vi "Planet_UserInterface.vi"(8 "error in":errorcluster, 9 "Number of it":i32, 11 "Conf":T1) -> (0 "error out":errorcluster, 3 "Exit?":bool)   [LabVIEW 2021]
uses:
  Typedefs/Axis.ctl
  Typedefs/ConfCluster.ctl
  Typedefs/All_Queues.ctl
  Typedefs/DataToUserInterface.ctl
  Typedefs/PropertyUserChange.ctl
  Typedefs/PropertiesRead_TDM.ctl
  Typedefs/Start_End.ctl
  Typedefs/OrderAnalysis.ctl
  Typedefs/MeassurementMode.ctl
  Typedefs/PropertiesOrderAnalysis.ctl
  Typedefs/AllDataToAnal.ctl
  Typedefs/PlanetInfo.ctl
  Typedefs/Detected peaks.ctl
  Typedefs/Referencias.ctl
  Typedefs/OpenClose.ctl
  Typedefs/DataToUI.ctl
  Typedefs/Results.ctl
panel:
  in  "Btn_Alarm":bool
  in  "Lock":bool
  in  "Stop":bool
  in  "Exit":bool
  in  "Btn_Mesh":bool
  in  "Btn_Order":bool
  in  "Btn_Spec":bool
  in  "Btn_Main":bool
  in  "Start":bool
  in  "Results":T6(tab)
  out "Vibration signals":waveform(dbl)[](graph)
  out "Speed profile":cluster{"time [s]":dbl[], "speed [RPM]":dbl[]}(graph)
  out "Input - Power Spectrum":cluster{"f0":dbl, "df":dbl, "magnitude":dbl[]}[](graph)
  out "Output - Power Spectrum":cluster{"f0":dbl, "df":dbl, "magnitude":dbl[]}[](graph)
  out "Input - Order power spectrum":T7(graph)
  out "Input - Actual max order":dbl
  out "Output - Order power spectrum":T7(graph)
  out "Output - Actual max order":dbl
  out "Input - fz":dbl[](graph) caption="Output - fz"
  out "Output_mean":dbl format="%0.2f"
  out "Output_std":dbl format="%0.2f"
  out "Input_mean":dbl format="%0.2f"
  out "WejścieInput":dbl format="%0.2f"
  out "Output - fz":dbl[](graph) caption="Input - fz"
  in  "Axis":T8 items=["X", "Y", "Z"]
  in  "Exceedances":i32(listbox)
  in  "MainSettings":enum32{"Page 1"}(tab)
  in  "averaging mode":u16(ring) items=["No averaging", "Vector averaging", "RMS averaging", "Peak hold"]
  in  "order resolution":dbl=0.1 min=0.0 format="%.3f"
  in  "window type":T9(ring)=enum."Hanning"
  in  "dB on":bool=TRUE
  in  "max order to analyze":dbl=32.0
  in  "Sample rate":i64=51200
  in  "File path":path
  in  "Channels":tag
  in  "Sample mode":i32(ring)=10123 items=["Finite Samples"=10178, "Continuous Samples"=10123, "Hardware Timed Single Point"=12522]
  in  "Terminal conf":i32(ring)=12529 items=["Default"=-1, "RSE"=10083, "NRSE"=10078, "Differential"=10106, "Pseudodifferential"=12529]
  in  "Multiple of Frequency":i32=3
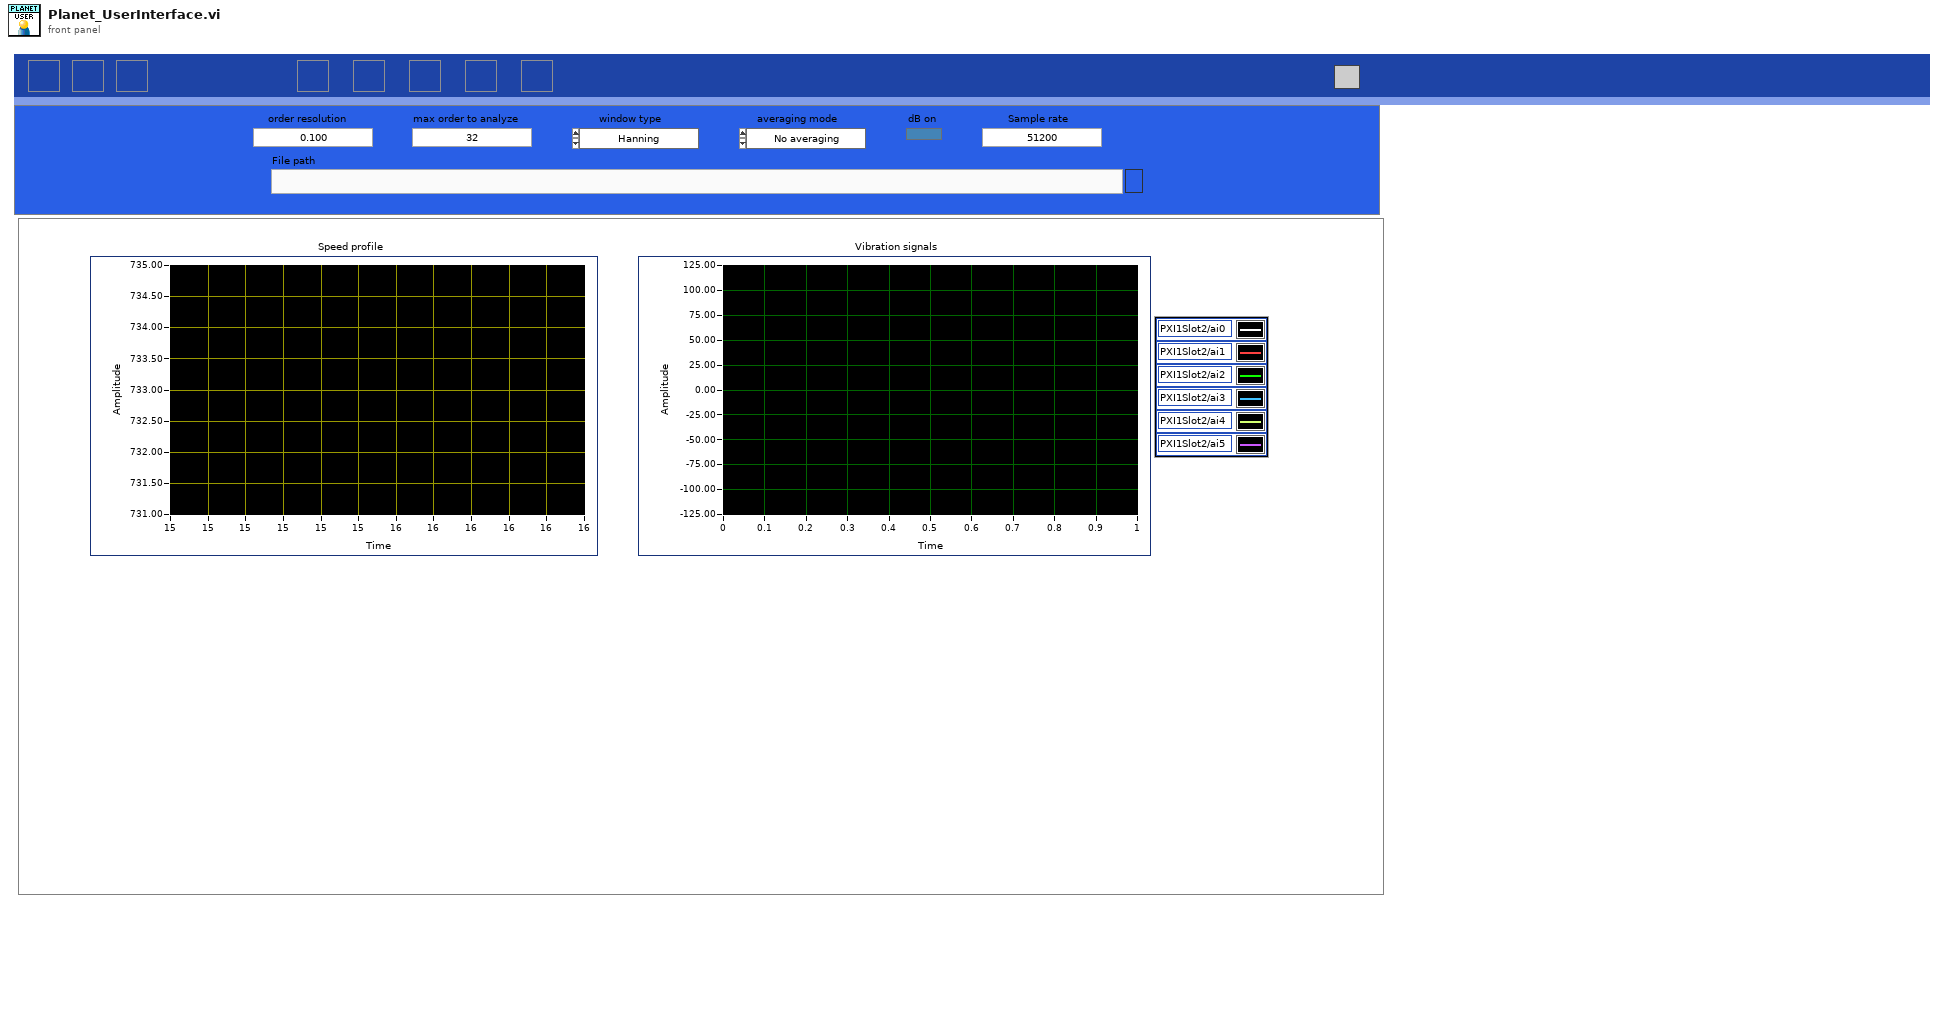
[diagram p1: front panel]
types:
  T1 = typedef "ConfCluster.ctl" = cluster{"Plik?":bool, "Queues":T2, "NewFile":path, "AllDataToAnal":T3}
  T2 = typedef "All_Queues.ctl" = cluster{"User Event":refnum<user-event>, "ToAcq":refnum<queue>, "ToOA":refnum<queue>}
  T3 = typedef "AllDataToAnal.ctl" = cluster{"PlanetInfo":T4, "Referencia":T5[][], "Ref?":bool}
  T4 = typedef "PlanetInfo.ctl" = cluster{"Ms":dbl, "Np":dbl, "Ns":dbl, "Nr":dbl}
  T5 = typedef "Detected peaks.ctl" = cluster{"detected frequency":dbl, "detected amplitude":dbl}
  T6 = enum32{"Main", "PowerSpectrum", "Order analysis", "Mesh Frequency", "Alarms"}
  T7 = cluster{"order 0":dbl, "delta order":dbl, "magnitude":dbl[]}[]
  T8 = typedef "Axis.ctl" = u16
  T9 = enum16{"None", "Hanning", "Hamming", "Blackman-Harris", "Exact Blackman", "Blackman", "Flat Top", "4 Term B-Harris", "7 Term B-Harris", "Low Sidelobe", "Gaussian"}
  T10 = typedef "Referencias.ctl" = cluster{"MainSettings":refnum<vi>, "Results":refnum<vi>, "FirstLineSettings":refnum<vi>[], "FromFile":refnum<vi>, "Meassurement":refnum<vi>[], "MainGraphs":refnum<vi>[], "OAGraphs":refnum<vi>[], "OA_MaxOrder":refnum<vi>[], "PSGraphs":refnum<vi>[], "Fz":refnum<vi>[], "mean_std":refnum<vi>[], "Btn":refnum<vi>[], "This VI":refnum<vi>, "Przekroczenia":refnum<vi>, "Axis":refnum<vi>, "Main_Btn":refnum<vi>[]}
  T11 = typedef "OpenClose.ctl" = enum16{"Close", "Open"}
  T12 = typedef "PropertiesRead_TDM.ctl" = cluster{"Start/End":T13, "stop":bool, "file path":path, "OrderAnalysis":T14, "Meassurement Mode":T15}
  T13 = typedef "Start_End.ctl" = enum16{"Start", "End"}
  T14 = typedef "OrderAnalysis.ctl" = cluster{"dB on":bool, "window type":u32, "max order to analyze":dbl, "order resolution":dbl, "Axis":T8, "Sample rate":i64, "Save?":bool, "Multiple_Frequency":i32, "averaging mode":enum16{"No averaging", "Vector averaging", "RMS averaging", "Peak hold"}}
  T15 = typedef "MeassurementMode.ctl" = cluster{"Sample mode":i32, "Terminal conf":i32, "Channels":tag}
  T16 = typedef "DataToUI.ctl" = cluster{"Speed profile":cluster{"time [s]":dbl[], "speed [RPM]":dbl[]}, "Results":T17[], "Vibration signals":waveform(dbl)[]}
  T17 = typedef "Results.ctl" = cluster{"Power Spectrum / PSD":cluster{"f0":dbl, "df":dbl, "magnitude":dbl[]}[], "Order power spectra":cluster{"order 0":dbl, "delta order":dbl, "magnitude":dbl[]}[], "Actual max order":dbl, "Mesh_Freq":dbl[], "Detected peaks":T5[][], "Alarm?":bool[], "Exceed":string[][], "Mesh_mean":dbl, "Mesh_std":dbl}
  T18 = typedef "PropertyUserChange.ctl" = enum16{"Default", "Results", "Start", "Save", "CanalNames"}
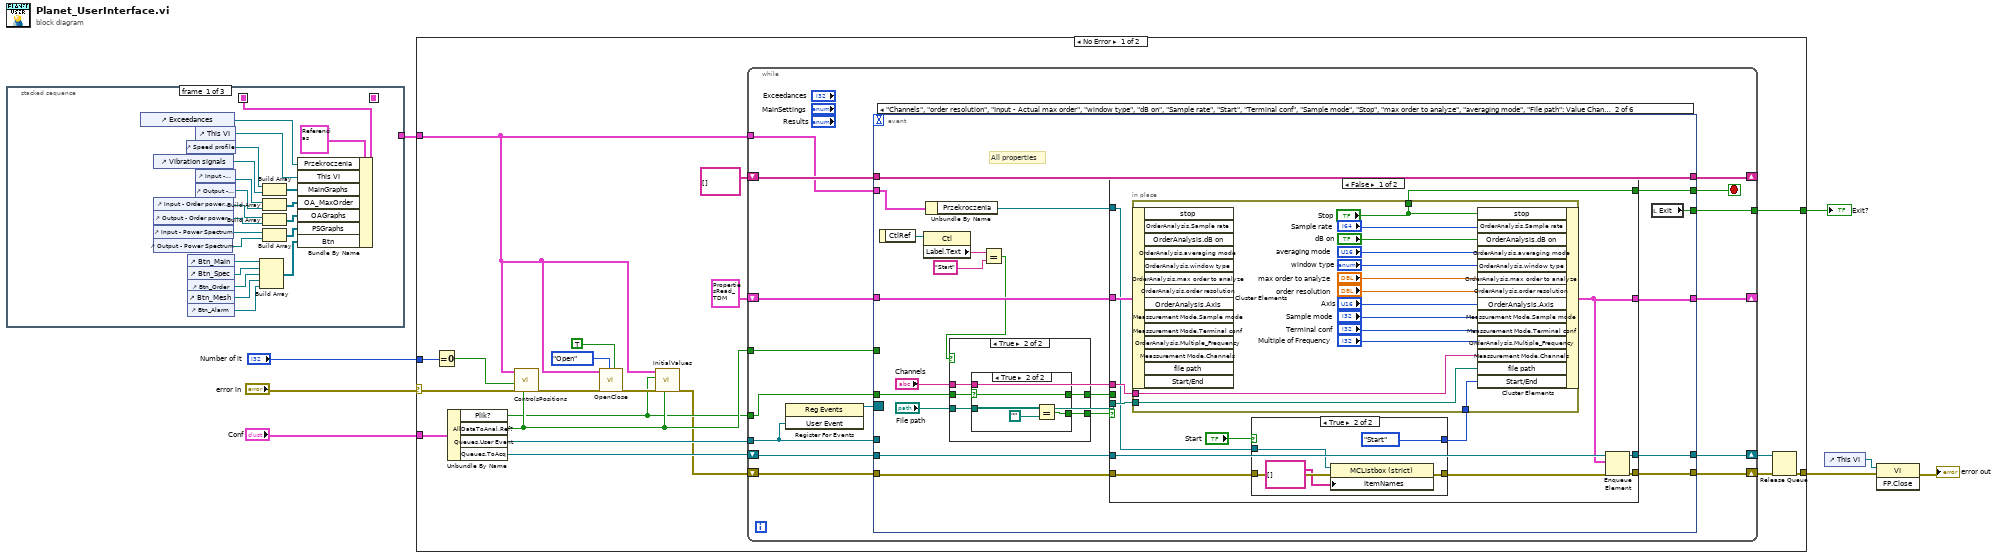
[diagram p0: block diagram]
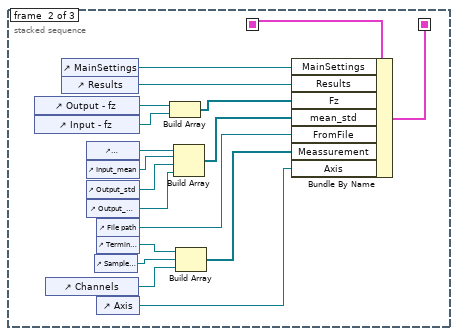
[diagram p2: hidden frame]
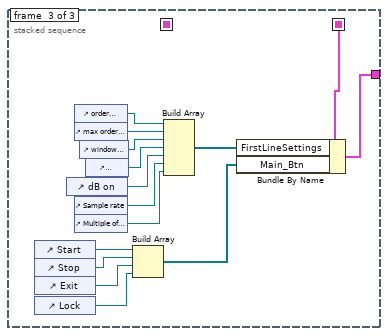
[diagram p3: hidden frame]
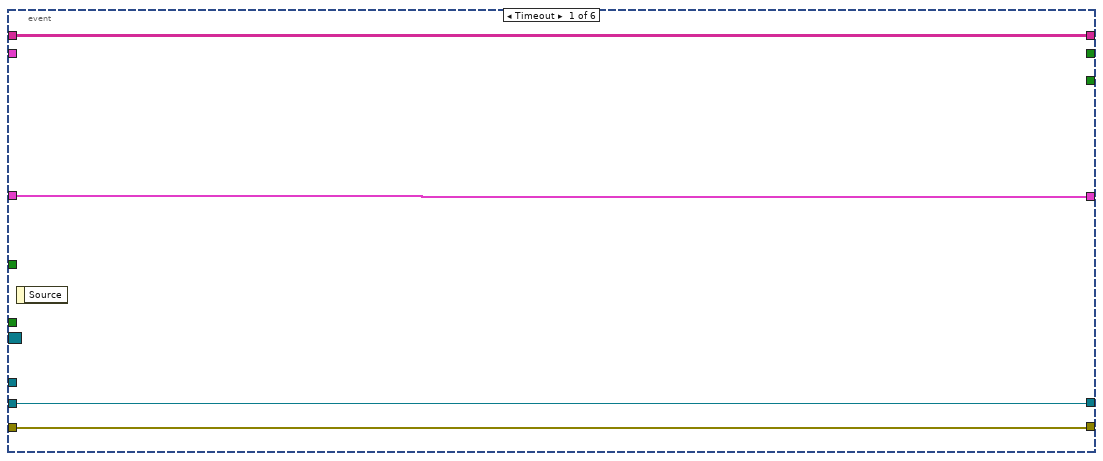
[diagram p4: hidden frame]
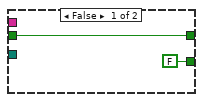
[diagram p5: hidden frame]
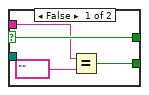
[diagram p6: hidden frame]
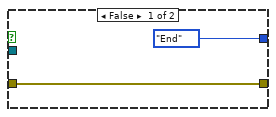
[diagram p7: hidden frame]
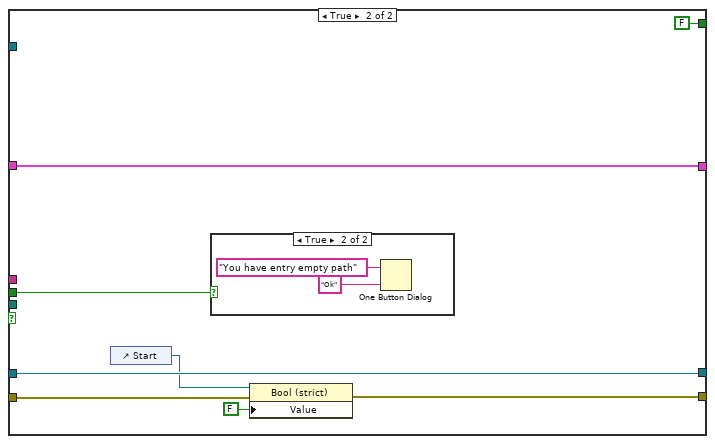
[diagram p8: hidden frame]
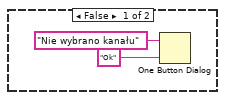
[diagram p9: hidden frame]
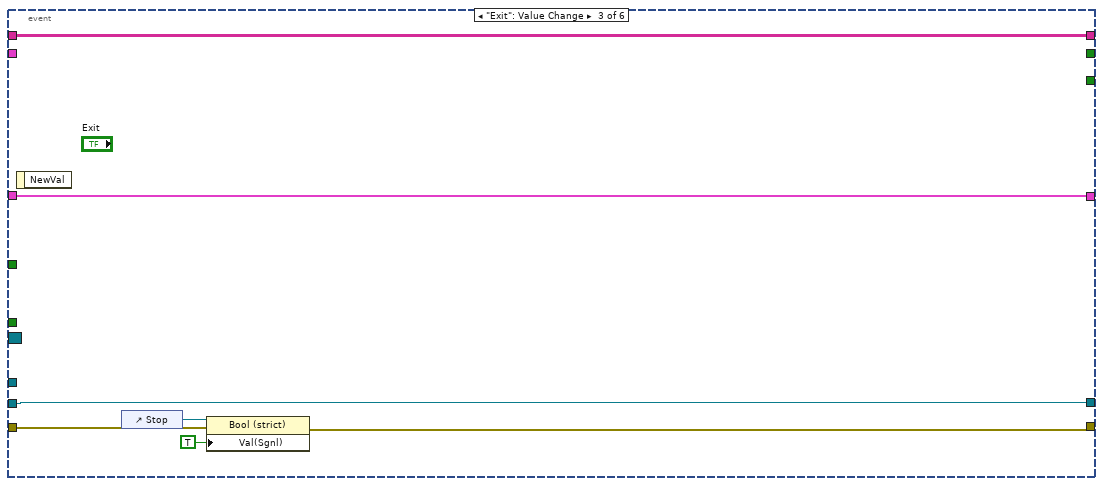
[diagram p10: hidden frame]
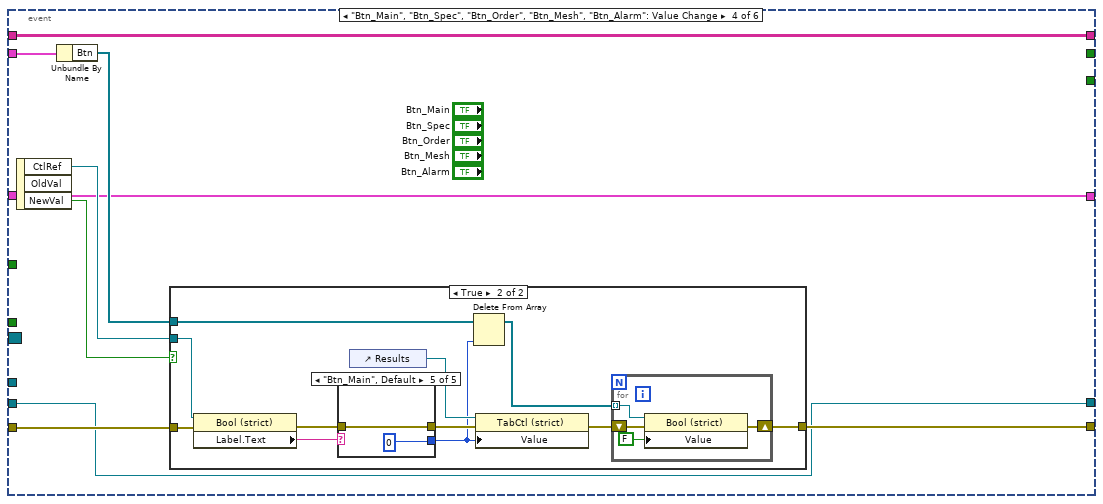
[diagram p11: hidden frame]
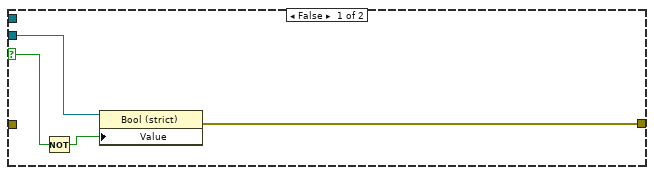
[diagram p12: hidden frame]
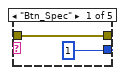
[diagram p13: hidden frame]
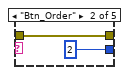
[diagram p14: hidden frame]
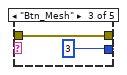
[diagram p15: hidden frame]
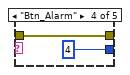
[diagram p16: hidden frame]
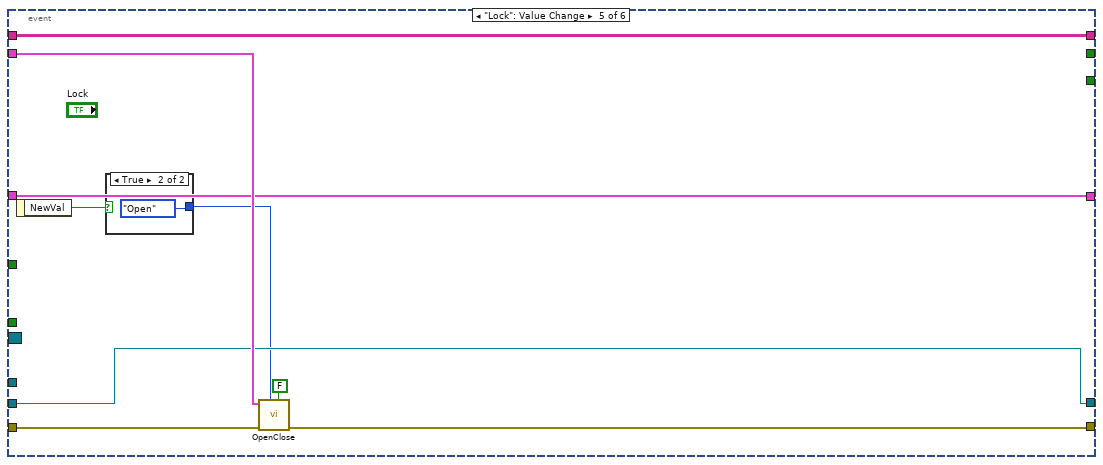
[diagram p17: hidden frame]
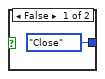
[diagram p18: hidden frame]
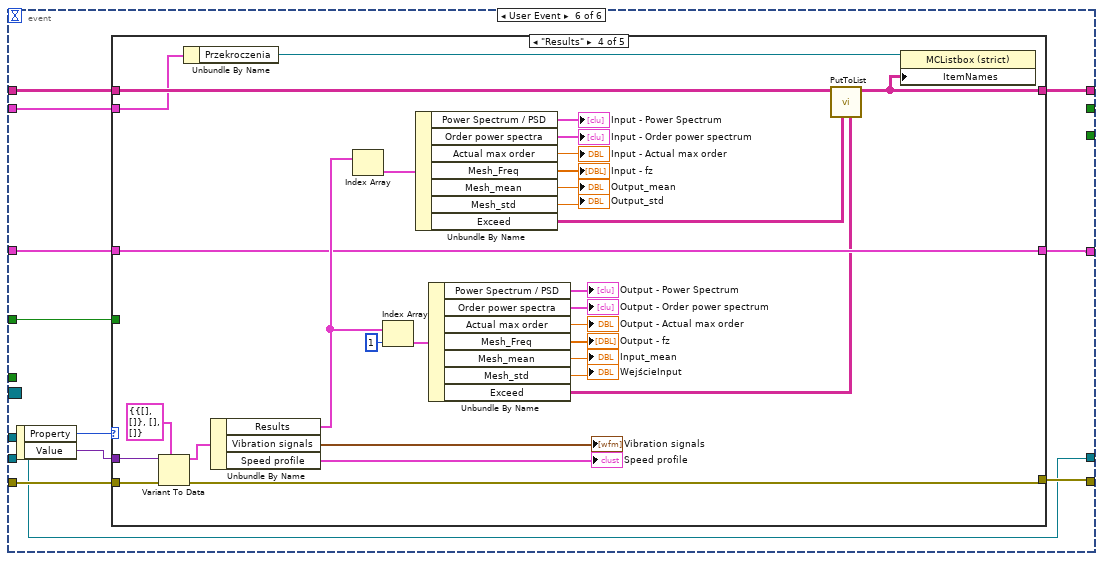
[diagram p19: hidden frame]
diagram:
  n1 = stacked-sequence {
    seq-local: [w15 _ _] -> [_ w33 _]
    seq-local: [_ w31 _] -> [_ _ w51]
    tunnel: [_ _ w50] -> w1
    frame #0 {
      n2 = control-ref of="Exceedances"() -> (w21:refnum<vi>)
      n3 = control-ref of="Output - Power Spectrum"() -> (w30:refnum<vi>)
      n4 = control-ref of="Vibration signals"() -> (w24:refnum<vi>)
      n5 = control-ref of="Input - Order power spectrum"() -> (w27:refnum<vi>)
      n6 = control-ref of="Output - Order power spectrum"() -> (w28:refnum<vi>)
      n7 = control-ref of="Input - Power Spectrum"() -> (w29:refnum<vi>)
      n8 = control-ref of="Speed profile"() -> (w23:refnum<vi>)
      n9 = control-ref of="Btn_Main"() -> (w10:refnum<vi>)
      n10 = control-ref of="Btn_Spec"() -> (w11:refnum<vi>)
      n11 = control-ref of="Btn_Order"() -> (w12:refnum<vi>)
      n12 = control-ref of="Btn_Mesh"() -> (w13:refnum<vi>)
      n13 = control-ref of="Btn_Alarm"() -> (w14:refnum<vi>)
      n14 = control-ref of="This VI"() -> (w20:refnum<vi>)
      n15 = control-ref of="Input - Actual max order"() -> (w25:refnum<vi>)
      n16 = control-ref of="Output - Actual max order"() -> (w26:refnum<vi>)
      n17 = Build Array(w10, w11, w12, w13, w14) -> (w9:refnum<vi>[])
      n18 = Build Array(w23, w24) -> (w19:refnum<vi>[])
      n19 = Build Array(w25, w26) -> (w18:refnum<vi>[])
      n20 = Build Array(w27, w28) -> (w17:refnum<vi>[])
      n21 = Build Array(w29, w30) -> (w16:refnum<vi>[])
      n22 = Bundle By Name(cluster=T10 {"MainSettings"=refnum, "Results"=refnum, "FirstLineSettings"=[], "FromFile"=refnum, "Meassurement"=[], "MainGraphs"=[], "OAGraphs"=[], "OA_MaxOrder"=[], "PSGraphs"=[], "Fz"=[], "mean_std"=[], "Btn"=[], "This VI"=refnum, "Przekroczenia"=refnum, "Axis"=refnum, "Main_Btn"=[]} ("References"), "Przekroczenia"=w21, "This VI"=w20, "MainGraphs"=w19, "OA_MaxOrder"=w18, "OAGraphs"=w17, "PSGraphs"=w16, "Btn"=w9) -> (w15:T10)
    }
    frame #1 {
      n23 = control-ref of="Output - fz"() -> (w48:refnum<vi>)
      n24 = control-ref of="Input - fz"() -> (w43:refnum<vi>)
      n25 = control-ref of="Channels"() -> (w40:refnum<vi>)
      n26 = control-ref of="MainSettings"() -> (w39:refnum<vi>)
      n27 = control-ref of="Results"() -> (w38:refnum<vi>)
      n28 = control-ref of="WejścieInput"() -> (w44:refnum<vi>)
      n29 = control-ref of="Input_mean"() -> (w45:refnum<vi>)
      n30 = control-ref of="Output_std"() -> (w46:refnum<vi>)
      n31 = control-ref of="Output_mean"() -> (w47:refnum<vi>)
      n32 = control-ref of="Sample mode"() -> (w42:refnum<vi>)
      n33 = control-ref of="File path"() -> (w35:refnum<vi>)
      n34 = control-ref of="Terminal conf"() -> (w41:refnum<vi>)
      n35 = control-ref of="Axis"() -> (w32:refnum<vi>)
      n36 = Build Array(w48, w43) -> (w37:refnum<vi>[])
      n37 = Build Array(w44, w45, w46, w47) -> (w36:refnum<vi>[])
      n38 = Build Array(w41, w42, w40) -> (w34:refnum<vi>[])
      n39 = Bundle By Name(cluster=w33, "MainSettings"=w39, "Results"=w38, "Fz"=w37, "mean_std"=w36, "FromFile"=w35, "Meassurement"=w34, "Axis"=w32) -> (w31:T10)
    }
    frame #2 {
      n40 = control-ref of="Start"() -> (w60:refnum<vi>)
      n41 = control-ref of="Stop"() -> (w61:refnum<vi>)
      n42 = control-ref of="Exit"() -> (w49:refnum<vi>)
      n43 = control-ref of="Lock"() -> (w62:refnum<vi>)
      n44 = control-ref of="dB on"() -> (w58:refnum<vi>)
      n45 = control-ref of="order resolution"() -> (w54:refnum<vi>)
      n46 = control-ref of="max order to analyze"() -> (w55:refnum<vi>)
      n47 = control-ref of="Sample rate"() -> (w59:refnum<vi>)
      n48 = control-ref of="Multiple of Frequency"() -> (w63:refnum<vi>)
      n49 = control-ref of="window type"() -> (w56:refnum<vi>)
      n50 = control-ref of="averaging mode"() -> (w57:refnum<vi>)
      n51 = Build Array(w60, w61, w49, w62) -> (w52:refnum<vi>[])
      n52 = Build Array(w54, w55, w56, w57, w58, w59, w63) -> (w53:refnum<vi>[])
      n53 = Bundle By Name(cluster=w51, "FirstLineSettings"=w53, "Main_Btn"=w52) -> (w50:T10)
    }
  }
  n54 = case shown="No Error" "error in" {
    selector: "error in" -> [w71 w338]
    tunnel: [w78 _] -> w8
    tunnel: "Conf" -> [w72 _]
    tunnel: [w70 w338] -> w5
    tunnel: "Number of it" -> [w65 _]
    tunnel: w1 -> [w67 _]
    frame No Error {
      n55 = Equal To 0?(x=w65) -> (x = 0?=w64:bool)
      n56 = Unbundle By Name(w72) -> ("Plik?"=w68:bool, "AllDataToAnal.Ref?"=w73:bool, "Queues.User Event"=w80:refnum<user-event>, "Queues.ToAcq"=w81:refnum<queue>)
      n57 = call "ControlsPositions.vi"("Ref?"=w73, "error in (no error)"=w71, "Boolean"=w64, "Referencia"=w67) -> ("error out"=w76:errorcluster)  [unwired: 7 in]
      n58 = call "OpenClose.vi"("FastOpen?"=TRUE, "Open/Close"=OpenClose."Open", "error in"=w76, "References"=w67) -> ("error out"=w75:errorcluster)  [unwired: 7 in]
      n59 = call "InitialValues.vi"("Ref?"=w73, "error in (no error)"=w75, "Plik?"=w68, "References"=w67) -> ("error out"=w66:errorcluster)  [unwired: 7 in]
      n60 = while {
        shift-right: [w94] -> w83
        shift-left: w81 -> [w96]
        shift-right: [w93] -> w82
        shift-left: w66 -> [w95]
        shift-right: [w97] -> _
        shift-left: T12 {"Start/End"=enum."End", "stop"=FALSE, "file path"=path "", "OrderAnalysis"={"dB on"=TRUE, "window type"=1, "max order to analyze"=32.0, "order resolution"=0.1, "Axis"=0, "Sample rate"=5000, "Save?"=FALSE, "Multiple_Frequency"=3, "averaging mode"=enum."No averaging"}, "Meassurement Mode"={"Sample mode"=10123, "Terminal conf"=12529, "Channels"=""}} -> [w98]
        tunnel: w80 -> [w90]
        tunnel: [w89] -> w78
        shift-right: [w87] -> _
        shift-left: string[][] [] ("Next") -> [w88]
        tunnel: w73 -> [w86]
        tunnel: w68 -> [w85]
        tunnel: w67 -> [w84]
        stop <- w92 stop-if-true
        n61 = register-events(w90) -> (reference out=w91:refnum<event-registration>)  [unwired: 2 in, 1 out]
        n62 = event shown="[1] \"Channels\", \"order resolution\", \"Input - Actual max order\", \"window type\", \"dB on\", \"Sample rate\", \"Start\", \"Terminal conf\", \"Sample mode\", \"Stop\", \"max order to analyze\", \"averaging mode\", \"File path\": Value Change" {
          selector: w91 -> [_ _ _ _ _ _]
          dyn-events: _ -> [_ _ _ _ _ _]
          timeout: _ -> [_ _ _ _ _ _]
          tunnel: w98 -> [w102 w122 w189 w193 w232 w245]
          tunnel: [w102 w117 w189 w193 w232 w244] -> w97
          tunnel: w96 -> [w101 w121 w187 w192 w233 w246]
          tunnel: w95 -> [w100 w120 w190 w194 w237 w249]
          tunnel: [w101 w119 w187 w192 w233 w246] -> w94
          tunnel: [w100 w118 w188 w195 w235 w248] -> w93
          tunnel: [_ w115 _ _ _ _] -> w92
          tunnel: w90 -> [_ _ _ _ _ _]
          tunnel: w84 -> [_ w108 _ w197 w236 w240]
          tunnel: [_ w114 _ _ _ _] -> w89
          tunnel: w88 -> [w99 w116 w184 w191 w229 w243]
          tunnel: [w99 w116 w184 w191 w229 w242] -> w87
          tunnel: w86 -> [_ _ _ _ _ w241]
          tunnel: w85 -> [_ w112 _ _ _ _]
          event Timeout {
            n63 = event-data() -> ()  [unwired: 1 in, 1 out]
          }
          event "Channels", "order resolution", "Input - Actual max order", "window type", "dB on", "Sample rate", "Start", "Terminal conf", "Sample mode", "Stop", "max order to analyze", "averaging mode", "File path": Value Change {
            # "All properties"
            n64 = event-data() -> ("CtlRef"=w106:refnum<vi>)  [unwired: 1 in]
            n65 = property class="Ctl"(reference=w106) -> ("Label.Text"=w105:string)  [unwired: 1 in, 2 out]
            n66 = Unbundle By Name(w108) -> ("Przekroczenia"=w107:refnum<vi>)
            n67 = Equal?(x=w105, y="Start") -> (x = y?=w103:bool)
            n68 = case shown="True" w103 {
              tunnel: [FALSE w129] -> w113
              tunnel: w112 -> [w124 w128]
              tunnel: "Channels" -> [_ w127]
              tunnel: "File path" -> [_ w126]
              tunnel: [w124 w125] -> w109
              frame False {
              }
              frame True {
                n69 = case shown="True" w128 {
                  selector: w128 -> [w133 w135]
                  tunnel: [w130 w136] -> w129
                  tunnel: w127 -> [w131 _]
                  tunnel: w126 -> [_ w134]
                  tunnel: [w133 w135] -> w125
                  frame False {
                    n70 = Equal?(x=w131, y=tag "" ("Channels")) -> (x = y?=w130:bool)
                  }
                  frame True {
                    n71 = Equal?(x=w134, y=path "") -> (x = y?=w136:bool)
                  }
                }
              }
            }
            n72 = case shown="False" w113 {
              tunnel: w122 -> [w150 w177]
              tunnel: w121 -> [w149 w178]
              tunnel: w120 -> [w140 w175]
              tunnel: [w148 w178] -> w119
              tunnel: [w147 w174] -> w118
              tunnel: [w146 w177] -> w117
              tunnel: [w143 FALSE ("Stop")] -> w115
              tunnel: "File path" -> [w142 _]
              tunnel: "Channels" -> [w141 _]
              tunnel: w109 -> [_ w176]
              tunnel: w107 -> [w138 _]
              frame False {
                n73 = case shown="True" "Start" {
                  tunnel: [Start_End."End" ("Start/End") Start_End."Start" ("Start/End")] -> w144
                  tunnel: w140 -> [w151 w156]
                  tunnel: [w151 w155] -> w139
                  tunnel: w138 -> [_ w153]
                  frame False {
                  }
                  frame True {
                    n74 = property class="MCListbox (strict)"(reference=w153, error in=w156, "ItemNames"=string[][] [] ("Next")) -> (error out=w155:errorcluster)  [unwired: 1 out]
                  }
                }
                n75 = in-place {
                  in-place-border: ["Stop"] -> w143
                  in-place-border: w144 -> [w165]
                  in-place-border: w142 -> [w160]
                  in-place-border: w141 -> [w158]
                  n76 = in-place-cluster #1(w150) -> ()  [unwired: 14 out]
                  n77 = in-place-cluster #1("stop"="Stop", "OrderAnalysis.Sample rate"="Sample rate", "OrderAnalysis.dB on"="dB on", "OrderAnalysis.averaging mode"="averaging mode", "OrderAnalysis.window type"="window type", "OrderAnalysis.max order to analyze"="max order to analyze", "OrderAnalysis.order resolution"="order resolution", "OrderAnalysis.Axis"="Axis", "Meassurement Mode.Sample mode"="Sample mode", "Meassurement Mode.Terminal conf"="Terminal conf", "OrderAnalysis.Multiple_Frequency"="Multiple of Frequency", "Meassurement Mode.Channels"=w158, "file path"=w160, "Start/End"=w165) -> (w146:T12)
                }
                n78 = Enqueue Element(queue=w149, element=w146, error in (no error)=w139) -> (queue out=w148:refnum<queue>, error out=w147:errorcluster)  [unwired: 1 in, 1 out]
              }
              frame True {
                n79 = control-ref of="Start"() -> (w173:refnum<vi>)
                n80 = case shown="True" w176 {
                  frame False {
                    n81 = One Button Dialog(message="Nie wybrano kanału", button name ("OK")="Ok") -> ()  [unwired: 1 out]
                  }
                  frame True {
                    n82 = One Button Dialog(message="You have entry empty path", button name ("OK")="Ok") -> ()  [unwired: 1 out]
                  }
                }
                n83 = property class="Bool (strict)"(reference=w173, error in=w175, "Value"=FALSE) -> (error out=w174:errorcluster)  [unwired: 1 out]
              }
            }
            n84 = local read "Exit"() -> (w114:bool)
          }
          event "Exit": Value Change {
            n85 = event-data() -> ()  [unwired: 1 in, 1 out]
            n86 = control-ref of="Stop"() -> (w186:refnum<vi>)
            n87 = property class="Bool (strict)"(reference=w186, error in=w190, "Val(Sgnl)"=TRUE ("Value (Signaling)")) -> (error out=w188:errorcluster)  [unwired: 1 out]
          }
          event "Btn_Main", "Btn_Spec", "Btn_Order", "Btn_Mesh", "Btn_Alarm": Value Change {
            n88 = event-data() -> ("CtlRef"=w199:refnum<vi>, "NewVal"=w198:bool)  [unwired: 1 in, 1 out]
            n89 = Unbundle By Name(w197) -> ("Btn"=w196:refnum<vi>[])
            n90 = case shown="True" w198 {
              selector: w198 -> [w201 _]
              tunnel: w199 -> [w203 w214]
              tunnel: [w202 w206] -> w195
              tunnel: w196 -> [_ w209]
              tunnel: w194 -> [_ w204]
              frame False {
                n91 = Not(x=w201) -> (.not. x?=w200:bool)
                n92 = property class="Bool (strict)"(reference=w203, "Value"=w200) -> (error out=w202:errorcluster)  [unwired: 1 in, 1 out]
              }
              frame True {
                n93 = property class="Bool (strict)"(reference=w214, error in=w204) -> (error out=w212:errorcluster, "Label.Text"=w213:string)  [unwired: 1 out]
                n94 = case shown="\"Btn_Main\", Default" w213 {
                  tunnel: w212 -> [w220 w222 w224 w226 w228]
                  tunnel: [w220 w222 w224 w226 w228] -> w211
                  tunnel: [1 2 3 4 0] -> w208
                  frame "Btn_Spec" {
                  }
                  frame "Btn_Order" {
                  }
                  frame "Btn_Mesh" {
                  }
                  frame "Btn_Alarm" {
                  }
                  frame "Btn_Main", Default {
                  }
                }
                n95 = control-ref of="Results"() -> (w210:refnum<vi>)
                n96 = Delete From Array(array=w209, index=w208) -> (array with subset deleted=w205:refnum<vi>[])  [unwired: 1 in, 1 out]
                n97 = property class="TabCtl (strict)"(reference=w210, error in=w211, "Value"=w208) -> (error out=w207:errorcluster)  [unwired: 1 out]
                n98 = for {
                  shift-right: [w216] -> w206
                  shift-left: w207 -> [w218]
                  tunnel: w205 -> [w217] mode=indexing
                  n99 = property class="Bool (strict)"(reference=w217, error in=w218, "Value"=FALSE) -> (error out=w216:errorcluster)  [unwired: 1 out]
                }
              }
            }
          }
          event "Lock": Value Change {
            n100 = event-data() -> ("NewVal"=w231:bool)  [unwired: 1 in]
            n101 = case shown="True" w231 {
              tunnel: [OpenClose."Close" ("Open/Close") OpenClose."Open" ("Open/Close")] -> w230
              frame False {
              }
              frame True {
              }
            }
            n102 = call "OpenClose.vi"("FastOpen?"=FALSE, "Open/Close"=w230, "error in"=w237, "References"=w236) -> ("error out"=w235:errorcluster)  [unwired: 7 in]
          }
          event User Event {
            n103 = event-data() -> ("Property"=w247:T18, "Value"=w250:variant)  [unwired: 1 in]
            n104 = case shown="\"Results\"" w247 {
              tunnel: w250 -> [_ w263 w284 w318 w334]
              tunnel: w249 -> [w253 w259 w285 w319 w335]
              tunnel: [w253 w258 w270 w312 w330] -> w248
              tunnel: w245 -> [w252 w257 w269 w311 w333]
              tunnel: [w252 w256 w269 w311 w332] -> w244
              tunnel: w243 -> [w251 w255 w268 w301 w329]
              tunnel: [w251 w255 w268 w304 w329] -> w242
              tunnel: w241 -> [_ w254 _ _ _]
              tunnel: w240 -> [_ _ _ w300 _]
              frame "Default", Default {
              }
              frame "Start" {
                n105 = Variant To Data(error in=w259, type=FALSE ("Parameters.Error?"), Variant=w263) -> (data=w260:bool, error out=w261:errorcluster)
                n106 = case shown="False" w254 {
                  tunnel: w257 -> [w265 w267]
                  tunnel: [w264 w267] -> w256
                  frame False {
                    n107 = in-place {
                      n108 = in-place-cluster #2(w265) -> ()  [unwired: 1 out]
                      n109 = in-place-cluster #2("OrderAnalysis.Save?"=TRUE) -> (w264:T12)
                    }
                  }
                  frame True {
                  }
                }
                n110 = property on="Start" class="Bool (strict)"(error in=w261, "Val(Sgnl)"=w260) -> (error out=w258:errorcluster)  [unwired: 1 in, 1 out]
              }
              frame "CanalNames" {
                n111 = Variant To Data(error in=w285, type=string[] [] ("deleted portion"), Variant=w284) -> (data=w278:string[], error out=w270:errorcluster)
                n112 = Delete From Array(array=w278, length=3, index=3) -> (deleted portion=w274:string[], array with subset deleted=w275:string[])
                n113 = control-ref of="Input - Power Spectrum"() -> (w281:refnum<vi>)
                n114 = control-ref of="Input - Order power spectrum"() -> (w280:refnum<vi>)
                n115 = control-ref of="Output - Power Spectrum"() -> (w273:refnum<vi>)
                n116 = control-ref of="Output - Order power spectrum"() -> (w272:refnum<vi>)
                n117 = control-ref of="Vibration signals"() -> (w282:refnum<vi>)
                n118 = Build Array(w281, w280) -> (w279:refnum<vi>[])
                n119 = Build Array(w273, w272) -> (w271:refnum<vi>[])
                n120 = for {
                  tunnel: w279 -> [w292] mode=indexing
                  tunnel: w275 -> [w291]
                  n121 = for {
                    tunnel: w292 -> [w294]
                    tunnel: w291 -> [w293] mode=indexing
                    i -> [w295]
                    n122 = property on="Property Node" class="WFGraph (strict)"(reference=w294, "Active Plot"=w295, "Plot.Plot Name"=w293) -> ()  [unwired: 1 in, 2 out]
                  }
                }
                n123 = for {
                  tunnel: w271 -> [w287] mode=indexing
                  tunnel: w274 -> [w286]
                  n124 = for {
                    tunnel: w287 -> [w289]
                    tunnel: w286 -> [w288] mode=indexing
                    i -> [w290]
                    n125 = property on="Property Node" class="WFGraph (strict)"(reference=w289, "Active Plot"=w290, "Plot.Plot Name"=w288) -> ()  [unwired: 1 in, 2 out]
                  }
                }
                n126 = for {
                  tunnel: w278 -> [w297] mode=indexing
                  tunnel: w282 -> [w296]
                  i -> [w298]
                  n127 = property on="Property Node" class="WFGraph (strict)"(reference=w296, "Active Plot"=w298, "Plot.Plot Name"=w297) -> ()  [unwired: 1 in, 2 out]
                }
              }
              frame "Results" {
                n128 = Variant To Data(error in=w319, type=T16 {"Speed profile"={"time [s]"=[], "speed [RPM]"=[]}, "Results"=[], "Vibration signals"=[]} ("DataToUI"), Variant=w318) -> (data=w316:T16, error out=w312:errorcluster)
                n129 = Unbundle By Name(w300) -> ("Przekroczenia"=w299:refnum<vi>)
                n130 = Unbundle By Name(w316) -> ("Results"=w313:T17[], "Vibration signals"=→"Vibration signals":waveform(dbl)[], "Speed profile"=→"Speed profile":cluster{"time [s]":dbl[], "speed [RPM]":dbl[]})
                n131 = Index Array(array=w313) -> (element=w328:T17)  [unwired: 1 in]
                n132 = Index Array(array=w313, index=1) -> (element=w324:T17)
                n133 = Unbundle By Name(w328) -> ("Power Spectrum / PSD"=→"Input - Power Spectrum":cluster{"f0":dbl, "df":dbl, "magnitude":dbl[]}[], "Order power spectra"=→"Input - Order power spectrum":T7, "Actual max order"=→"Input - Actual max order":dbl, "Mesh_Freq"=→"Input - fz":dbl[], "Mesh_mean"=→"Output_mean":dbl, "Mesh_std"=→"Output_std":dbl, "Exceed"=w302:string[][])
                n134 = Unbundle By Name(w324) -> ("Power Spectrum / PSD"=→"Output - Power Spectrum":cluster{"f0":dbl, "df":dbl, "magnitude":dbl[]}[], "Order power spectra"=→"Output - Order power spectrum":T7, "Actual max order"=→"Output - Actual max order":dbl, "Mesh_Freq"=→"Output - fz":dbl[], "Mesh_mean"=→"Input_mean":dbl, "Mesh_std"=→"WejścieInput":dbl, "Exceed"=w303:string[][])
                n135 = call "PutToList.vi"("Wyjście_Exceed"=w303, "Wejscie_Exceed"=w302, "Previous"=w301) -> ("Next"=w304:string[][])  [unwired: 8 in]
                n136 = property class="MCListbox (strict)"(reference=w299, "ItemNames"=w304) -> ()  [unwired: 1 in, 2 out]
              }
              frame "Save" {
                n137 = Variant To Data(error in=w335, type=FALSE ("Parameters.Error?"), Variant=w334) -> (data=w331:bool, error out=w330:errorcluster)
                n138 = in-place {
                  in-place-border: w331 -> [w337]
                  n139 = in-place-cluster #3(w333) -> ()  [unwired: 1 out]
                  n140 = in-place-cluster #3("OrderAnalysis.Save?"=w337) -> (w332:T12)
                }
              }
            }
          }
        }
      }
      n141 = Release Queue(queue=w83, error in (no error)=w82) -> (error out=w70:errorcluster)  [unwired: 1 in, 2 out]
    }
    frame Error {
    }
  }
  "Exit?" <- w8
  n142 = control-ref of="This VI"() -> (w3:refnum<vi>)
  n143 = invoke class="VI" method="FP.Close"(reference=w3, error in=w5) -> (error out=→"error out":errorcluster)  [unwired: 1 in, 2 out]
